vi "Autonomous Independent.vi"() -> ()   [LabVIEW 2019]
doc: "This VI is called when autonomous begins, and will automatically be terminated when autonomous ends. You can carry out timed or sensor driven robot movement independently without needing to return to the caller."
uses:
  <vilib>/Rock Robotics/WPI/Ultrasonic/WPI_UltrasonicRangeUnits.ctl
  <vilib>/Rock Robotics/WPI/Utilities/WPI_GetSetVariantRefNum.vi
  <vilib>/Rock Robotics/Network Tables/NT Read String.vi
  <vilib>/Rock Robotics/Network Tables/NT Write Numeric Array.vi
  <vilib>/Rock Robotics/WPI/Ultrasonic/WPI_SonarSRF04DigitalRefNum Registry Get.vi
  <vilib>/Rock Robotics/WPI/Ultrasonic/WPI_SonarSRF04DigitalGetRange.vi
panel:
  out "Ultrasonic 3":dbl
  out "Ultrasonic 2":dbl
  out "Ultrasonic":dbl
  out "Degrees 2":dbl(knob) scale=0.0..360.0
  out "Degrees":dbl(knob) scale=0.0..360.0
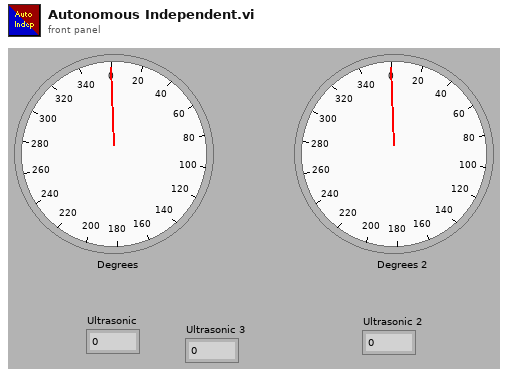
[diagram p1: front panel]
types:
  T1 = typedef "WPI_JoystickDevRef.ctl" = cluster{"Device":T2}
  T2 = typedef "WPI_JoystickDeviceEnum.ctl" = enum16{"USB 0", "USB 1", "USB 2", "USB 3", "USB 4", "USB 5"}
  T3 = typedef "WPI_UltrasonicRangeUnits.ctl" = enum16{"inches", "mm"}
  T4 = typedef "WPI_RobotDriveDevRef.ctl" = cluster{"DevStatus":errorcluster, "Motors[]":T5[], "Square Inputs":bool, "Max Output":dbl}
  T5 = typedef "WPI_MotorControlDeviceRef.ctl" = cluster{"DeviceStatus":errorcluster, "Type":T6, "PWM":cluster{"PWM Channel":T7, "DeadBand":T8}, "CAN":cluster{"Device Number":u8, "SetOutput VI Ref":variant, "GetOutput VI Ref":variant, "Enable VI Ref":variant, "Disable VI Ref":variant, "Data":variant}, "Invert":bool, "DIO PWM":cluster{"PWM \"Enable\" Channel":T7, "DIOChannel":T9, "PWM Rate":dbl}}
  T6 = typedef "WPI_MotorControlType.ctl" = enum16{"PWM", "CAN", "DIO PWM"}
  T7 = typedef "FPGA_DIOPWMChannel.ctl" = enum8{"PWM 0", "PWM 1", "PWM 2", "PWM 3", "PWM 4", "PWM 5", "PWM 6", "PWM 7", "PWM 8", "PWM 9", "PWM MXP 0", "PWM MXP 1", "PWM MXP 2", "PWM MXP 3", "PWM MXP 4", "PWM MXP 5", "PWM MXP 6", "PWM MXP 7", "PWM MXP 8", "PWM MXP 9", "Invalid"}
  T8 = typedef "WPI_PWMDeadband.ctl" = cluster{"Name":string, "maxPositivePwm":i32, "minPositivePwm":i32, "centerPwm":i32, "maxNegativePwm":i32, "minNegativePwm":i32, "angularRange":u16}
  T9 = typedef "FPGA_DIOChannel.ctl" = enum8{"DIO 0", "DIO 1", "DIO 2", "DIO 3", "DIO 4", "DIO 5", "DIO 6", "DIO 7", "DIO 8", "DIO 9", "DIO MXP 0", "DIO MXP 1", "DIO MXP 2", "DIO MXP 3", "DIO MXP 4", "DIO MXP 5", "DIO MXP 6", "DIO MXP 7", "DIO MXP 8", "DIO MXP 9", "DIO MXP 10", "DIO MXP 11", "DIO MXP 12", "DIO MXP 13", "DIO MXP 14", "DIO MXP 15", "SPI Port CS1", "SPI Port CS2", "SPI Port CS3", "SPI Port MISO", "SPI Port MOSI", "Invalid"}
  T10 = typedef "WPI_I2CDevRef.ctl" = cluster{"DevStatus":errorcluster, "Device Address":u8, "Handle":i32, "I2C Bus":T11}
  T11 = typedef "i2c_bus.ctl" = enum16{"I2C On-Board", "I2C MXP", "Invalid"}
  T12 = typedef "WPI_UltrasonicDeviceRef.ctl" = cluster{"DevStatus":errorcluster, "Ping Channel":T9, "Echo Channel":T9, "CntIndex":T13}
  T13 = typedef "FPGA_CounterCtrSystemIndex.ctl" = enum8{"Ctr 0", "Ctr 1", "Ctr 2", "Ctr 3", "Ctr 4", "Ctr 5", "Ctr 6", "Ctr 7", "Invalid"}
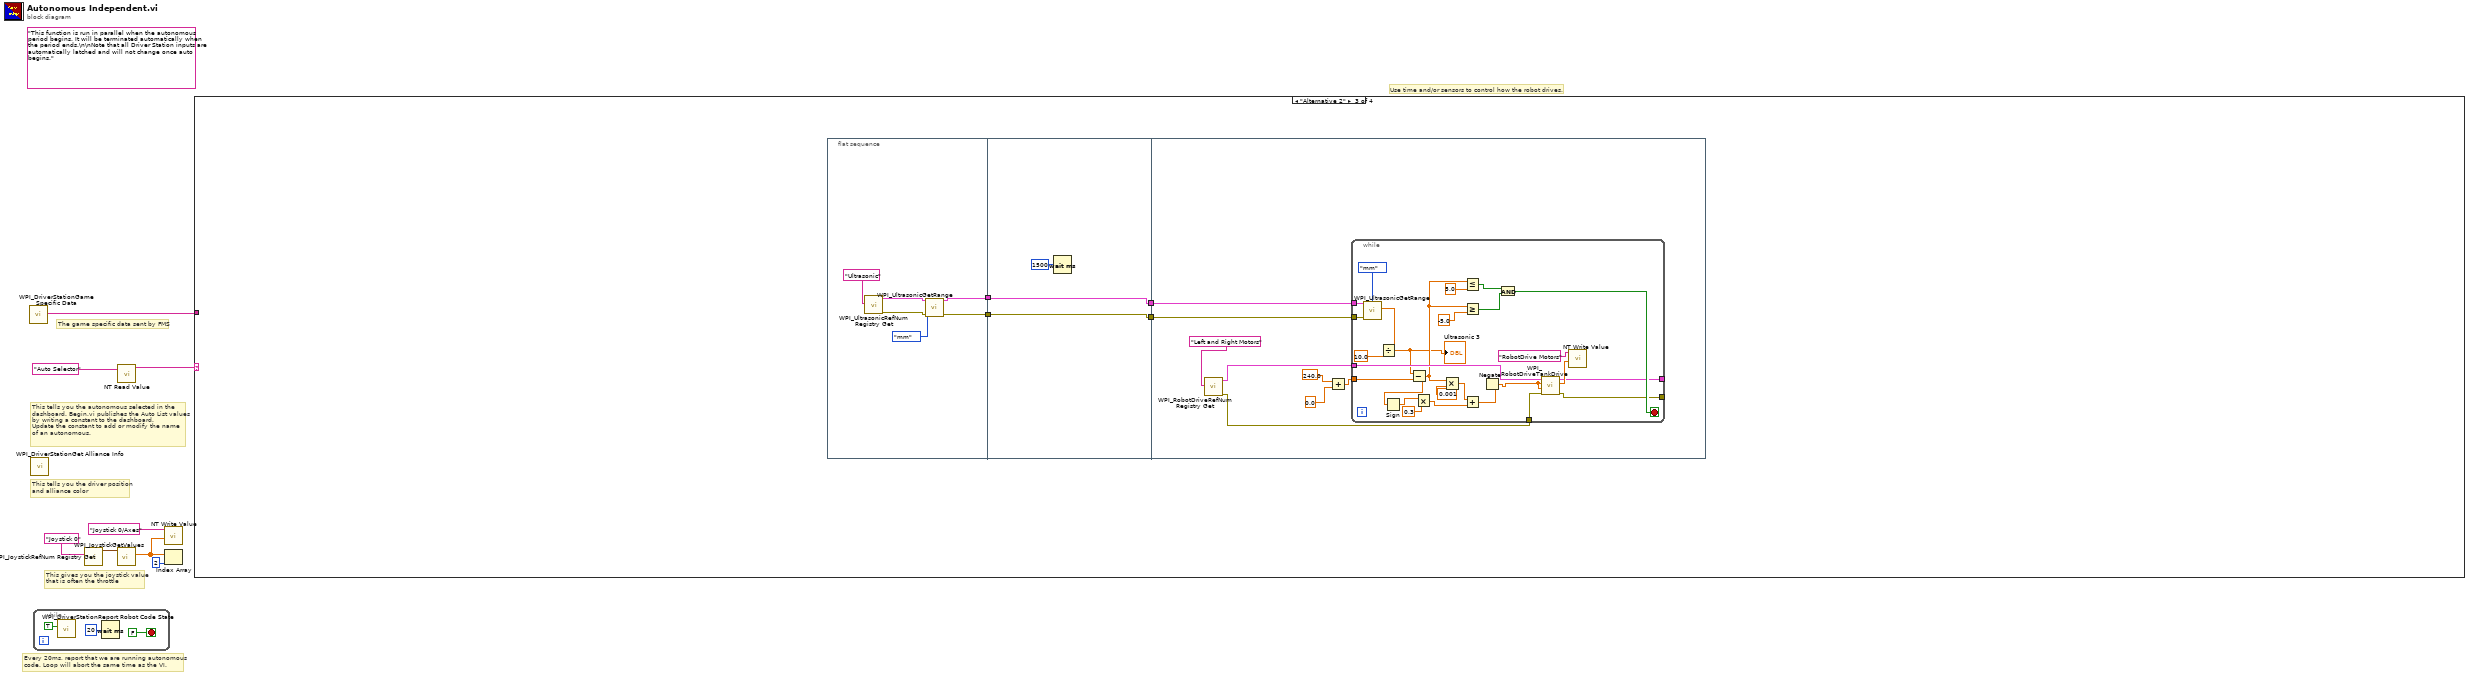
[diagram p0: block diagram]
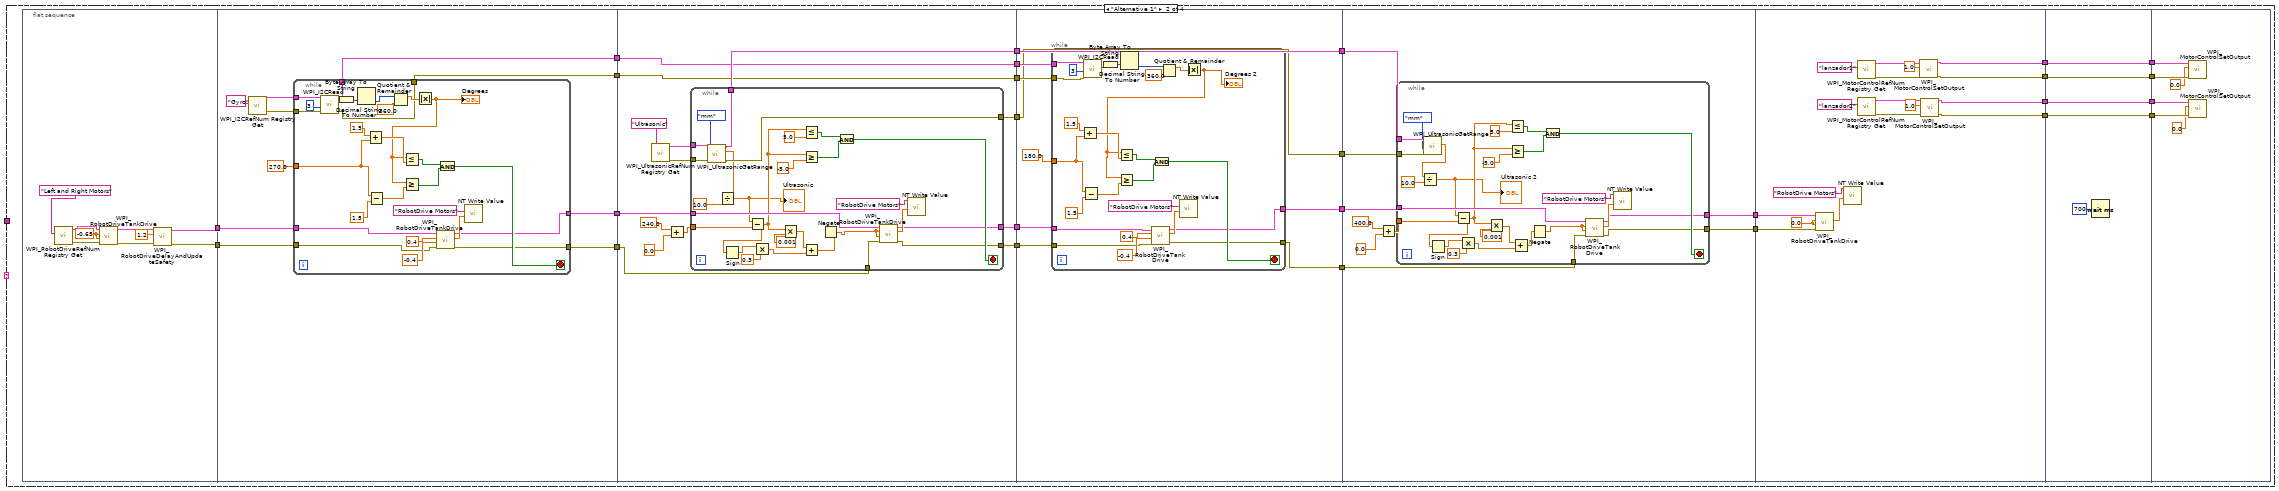
[diagram p3: hidden frame]
diagram:
  (unwired) "This function is run in parallel when the autonomous period begins. It will be terminated automatically when the period ends.\n\nNote that all Driver Station inputs are automatically latched and will not change once auto begins."
  # "The game specific data sent by FMS"
  # "This tells you the autonomous selected in the \ndashboard. Begin.vi publishes the Auto List values\nby writing a constant to the dashboard.\nUpdate the constant to add or modify the name\nof an autonomous."
  # "Every 20ms, report that we are running autonomous\ncode. Loop will abort the same time as the VI."
  # "This gives you the joystick value\nthat is often the throttle"
  # "Use time and/or sensors to control how the robot drives."
  # "This tells you the driver position\nand alliance color"
  n1 = call <vilib>:"WPI_DriverStationGame Specific Data.vi"() -> ("Game Specific Data"=w1:string)  [unwired: 11 in]
  n2 = call <vilib>:"WPI_DriverStationGet Alliance Info.vi"() -> ()  [unwired: 12 out]
  n3 = while {
    stop <- FALSE stop-if-true
    n4 = call <vilib>:"WPI_DriverStationReport Robot Code State.vi"("Autonomous"=TRUE) -> ()  [unwired: 10 in, 1 out]
    n5 = Wait (ms)(milliseconds to wait=u32 20) -> ()  [unwired: 1 out]
  }
  n6 = call <vilib>:"WPI_JoystickRefNum Registry Get.vi"("refnum name"="Joystick 0") -> ("JoystickDevRef"=w7:T1)  [unwired: 1 in, 9 out]
  n7 = call <vilib>:"WPI_JoystickGetValues.vi"("JoystickDevRef"=w7) -> ("Axes"=w3:dbl[])  [unwired: 6 in, 4 out]
  n8 = call-poly <vilib>:"NT Read Value.vi"("Name"="Auto Selector") -> ("String"=w4:string)  [unwired: 9 in, 1 out]
  n9 = call-poly <vilib>:"NT Write Value.vi"("Numeric Array"=w3, "Name"="Joystick 0/Axes") -> ()  [unwired: 9 in, 1 out]
  n10 = Index Array(array=w3, index=2) -> ()  [unwired: 1 out]
  n11 = case shown="\"Alternative 2\"" w4 {
    tunnel: w1 -> [_ _ _ _]
    frame Default {
      # "You can put your main auto here, or you can right-click on the case and make any\nother frame be the default case."
      # "This is the frame that will execute if no selection is made, or if it is not recognized"
    }
    frame "Alternative 1" {
      n12 = flat-sequence {
        tunnel: [w39] -> w15
        tunnel: [w40] -> w14
        tunnel: [w55] -> w37
        tunnel: [w54] -> w36
        tunnel: w15 -> [w50]
        tunnel: w14 -> [w49]
        tunnel: [w48] -> w13
        tunnel: [w47] -> w12
        tunnel: w37 -> [w91]
        tunnel: w36 -> [w90]
        tunnel: [w89] -> w35
        tunnel: [w88] -> w34
        tunnel: [w85] -> w33
        tunnel: [w84] -> w32
        tunnel: [w87] -> w31
        tunnel: [w86] -> w30
        tunnel: w13 -> [w85]
        tunnel: w12 -> [w84]
        tunnel: w35 -> [w134]
        tunnel: w34 -> [w133]
        tunnel: w33 -> [w131]
        tunnel: w32 -> [w130]
        tunnel: [w129] -> w29
        tunnel: [w128] -> w28
        tunnel: [w127] -> w27
        tunnel: w31 -> [w127]
        tunnel: [w126] -> w26
        tunnel: w30 -> [w126]
        tunnel: w29 -> [w168]
        tunnel: w28 -> [w164]
        tunnel: w27 -> [w163]
        tunnel: w26 -> [w162]
        tunnel: [w161] -> w25
        tunnel: [w160] -> w24
        tunnel: w25 -> [w201]
        tunnel: w24 -> [w200]
        tunnel: [w198] -> w23
        tunnel: [w197] -> w22
        tunnel: [w196] -> w21
        tunnel: [w195] -> w20
        tunnel: [w215] -> w19
        tunnel: w23 -> [w215]
        tunnel: [w214] -> w18
        tunnel: w22 -> [w214]
        tunnel: [w213] -> w17
        tunnel: w21 -> [w213]
        tunnel: [w212] -> w16
        tunnel: w20 -> [w212]
        tunnel: w19 -> [w222]
        tunnel: w18 -> [w221]
        tunnel: w17 -> [w220]
        tunnel: w16 -> [w219]
        frame #0 {
          w44 = -0.65 ("Left axis value")
          n13 = call <vilib>:"WPI_RobotDriveRefNum Registry Get.vi"("refnum name"="Left and Right Motors") -> ("error out"=w42:errorcluster, "RobotDriveDevRef"=w43:T4)  [unwired: 9 in]
          n14 = call <vilib>:"WPI_RobotDriveTankDrive.vi"("error in (no error)"=w42, "Right axis value"=w44, "Left axis value"=w44, "RobotDriveDevRef"=w43) -> ("error out"=w45:errorcluster, "RobotDriveDevRef"=w46:T4)  [unwired: 5 in, 1 out]
          n15 = call <vilib>:"WPI_RobotDriveDelayAndUpdateSafety.vi"("error in (no error)"=w45, "Delay (s)"=1.2, "RobotDriveDevRef"=w46) -> ("error out"=w39:errorcluster, "RobotDriveDevRef 2"=w40:T4)  [unwired: 7 in]
        }
        frame #1 {
          n16 = call <vilib>:"WPI_I2CRefNum Registry Get.vi"("refnum name"="Gyro") -> ("error out"=w52:errorcluster, "I2CDevRef"=w51:T10)  [unwired: 9 in]
          n17 = while {
            tunnel: 270.0 ("y") -> [w76]
            tunnel: [w69] -> w55
            tunnel: [w68] -> w54
            tunnel: w52 -> [w65]
            tunnel: w51 -> [w64]
            tunnel: w50 -> [w60]
            tunnel: w49 -> [w59]
            tunnel: [w58] -> w48
            tunnel: [w57] -> w47
            stop <- w79 stop-if-true
            n18 = call <vilib>:"WPI_I2CRead.vi"("error in (no error)"=w65, "I2CBytesToRead"=u8 3, "I2CDevRef"=w64) -> ("error out"=w57:errorcluster, "Data Out"=w62:u8[], "I2CDevRef"=w58:T10)  [unwired: 6 in]
            n19 = Byte Array To String(unsigned byte array=w62) -> (string=w66:string)
            n20 = Decimal String To Number(string=w66) -> (number=w61:i32)  [unwired: 2 in, 1 out]
            n21 = Add(x=1.5 ("y"), y=w76) -> (x+y=w72:dbl)
            n22 = Subtract(x=w76, y=1.5 ("x")) -> (x-y=w73:dbl)
            n23 = Quotient & Remainder(x=w61, y=360.0) -> (x-y*floor(x/y)=w70:dbl)  [unwired: 1 out]
            n24 = Absolute Value(x=w70) -> (abs(x)=w67:dbl)
            "Degrees" <- w67
            n25 = Less Or Equal?(x=w67, y=w72) -> (x <= y?=w74:bool)
            n26 = Greater Or Equal?(x=w67, y=w73) -> (x >= y?=w75:bool)
            n27 = call <vilib>:"WPI_RobotDriveTankDrive.vi"("error in (no error)"=w60, "Right axis value"=-0.4 ("X axis value"), "Left axis value"=0.4 ("X axis value"), "RobotDriveDevRef"=w59) -> ("error out"=w68:errorcluster, "Motor Values"=w83:dbl[], "RobotDriveDevRef"=w69:T4)  [unwired: 5 in]
            n28 = And(x=w74, y=w75) -> (x .and. y?=w79:bool)
            n29 = call-poly <vilib>:"NT Write Value.vi"("Numeric Array"=w83, "Name"="RobotDrive Motors") -> ()  [unwired: 9 in, 1 out]
          }
        }
        frame #2 {
          n30 = call-poly <vilib>:"WPI_UltrasonicRefNum Registry Get.vi"("refnum name"="Ultrasonic") -> ("error out"=w96:errorcluster, "SonarSRF04DevRef"=w95:T12)  [unwired: 9 in]
          n31 = Add(x=240.0 ("y"), y=0.0) -> (x+y=w92:dbl)
          n32 = while {
            tunnel: w96 -> [w107]
            tunnel: w95 -> [w106]
            tunnel: w92 -> [w125]
            tunnel: w91 -> [w120]
            tunnel: w90 -> [w116]
            tunnel: [w109] -> w89
            tunnel: [w108] -> w88
            tunnel: [w104] -> w87
            tunnel: [w103] -> w86
            stop <- w113 stop-if-true
            n33 = call-poly <vilib>:"WPI_UltrasonicGetRange.vi"("error in (no error)"=w107, "Range Units"=WPI_UltrasonicRangeUnits."mm", "SonarSRF04DevRef"=w106) -> ("error out"=w103:errorcluster, "Distance"=w102:dbl, "SonarSRF04DevRef"=w104:T12)  [unwired: 6 in]
            n34 = Divide(x=w102, y=10.0) -> (x/y=w100:dbl)
            "Ultrasonic" <- w100
            n35 = Subtract(x=w100, y=w125) -> (x-y=w110:dbl)
            n36 = Sign(1:w110) -> (0:w119:dbl)
            n37 = Multiply(x=w119, y=0.3) -> (x*y=w117:dbl)
            n38 = Multiply(x=w110, y=0.001) -> (x*y=w123:dbl)
            n39 = Less Or Equal?(x=w110, y=5.0 ("x")) -> (x <= y?=w115:bool)
            n40 = Greater Or Equal?(x=w110, y=-5.0 ("x")) -> (x >= y?=w114:bool)
            n41 = Add(x=w123, y=w117) -> (x+y=w99:dbl)
            n42 = Negate(x=w99) -> (-x=w98:dbl)
            n43 = And(x=w115, y=w114) -> (x .and. y?=w113:bool)
            n44 = call <vilib>:"WPI_RobotDriveTankDrive.vi"("error in (no error)"=w116, "Right axis value"=w98, "Left axis value"=w98, "RobotDriveDevRef"=w120) -> ("error out"=w109:errorcluster, "Motor Values"=w122:dbl[], "RobotDriveDevRef"=w108:T4)  [unwired: 5 in]
            n45 = call-poly <vilib>:"NT Write Value.vi"("Numeric Array"=w122, "Name"="RobotDrive Motors") -> ()  [unwired: 9 in, 1 out]
          }
        }
        frame #3 {
          n46 = while {
            tunnel: w133 -> [w155]
            tunnel: w134 -> [w154]
            tunnel: 180.0 ("y") -> [w150]
            tunnel: [w143] -> w129
            tunnel: [w142] -> w128
            tunnel: w131 -> [w138]
            tunnel: w130 -> [w137]
            stop <- w153 stop-if-true
            n47 = Add(x=1.5 ("y"), y=w150) -> (x+y=w146:dbl)
            n48 = Subtract(x=w150, y=1.5 ("x")) -> (x-y=w147:dbl)
            n49 = call <vilib>:"WPI_I2CRead.vi"("error in (no error)"=w137, "I2CBytesToRead"=u8 3, "I2CDevRef"=w138) -> ("Data Out"=w139:u8[])  [unwired: 6 in, 2 out]
            n50 = Byte Array To String(unsigned byte array=w139) -> (string=w141:string)
            n51 = Decimal String To Number(string=w141) -> (number=w136:i32)  [unwired: 2 in, 1 out]
            n52 = call <vilib>:"WPI_RobotDriveTankDrive.vi"("error in (no error)"=w154, "Right axis value"=-0.4 ("X axis value"), "Left axis value"=0.4 ("X axis value"), "RobotDriveDevRef"=w155) -> ("error out"=w142:errorcluster, "Motor Values"=w159:dbl[], "RobotDriveDevRef"=w143:T4)  [unwired: 5 in]
            n53 = Quotient & Remainder(x=w136, y=360.0) -> (x-y*floor(x/y)=w144:dbl)  [unwired: 1 out]
            n54 = call-poly <vilib>:"NT Write Value.vi"("Numeric Array"=w159, "Name"="RobotDrive Motors") -> ()  [unwired: 9 in, 1 out]
            n55 = Absolute Value(x=w144) -> (abs(x)=w135:dbl)
            "Degrees 2" <- w135
            n56 = Less Or Equal?(x=w135, y=w146) -> (x <= y?=w148:bool)
            n57 = Greater Or Equal?(x=w135, y=w147) -> (x >= y?=w149:bool)
            n58 = And(x=w148, y=w149) -> (x .and. y?=w153:bool)
          }
        }
        frame #4 {
          n59 = Add(x=400.0 ("y"), y=0.0) -> (x+y=w165:dbl)
          n60 = while {
            tunnel: w162 -> [w176]
            tunnel: w163 -> [w175]
            tunnel: w165 -> [w194]
            tunnel: w168 -> [w189]
            tunnel: w164 -> [w185]
            tunnel: [w178] -> w161
            tunnel: [w177] -> w160
            stop <- w182 stop-if-true
            n61 = call-poly <vilib>:"WPI_UltrasonicGetRange.vi"("error in (no error)"=w176, "Range Units"=WPI_UltrasonicRangeUnits."mm", "SonarSRF04DevRef"=w175) -> ("Distance"=w173:dbl)  [unwired: 6 in, 2 out]
            n62 = Divide(x=w173, y=10.0) -> (x/y=w171:dbl)
            "Ultrasonic 2" <- w171
            n63 = Subtract(x=w171, y=w194) -> (x-y=w179:dbl)
            n64 = Sign(1:w179) -> (0:w188:dbl)
            n65 = Multiply(x=w188, y=0.3) -> (x*y=w186:dbl)
            n66 = Multiply(x=w179, y=0.001) -> (x*y=w192:dbl)
            n67 = Less Or Equal?(x=w179, y=5.0 ("x")) -> (x <= y?=w184:bool)
            n68 = Greater Or Equal?(x=w179, y=-5.0 ("x")) -> (x >= y?=w183:bool)
            n69 = Add(x=w192, y=w186) -> (x+y=w170:dbl)
            n70 = Negate(x=w170) -> (-x=w169:dbl)
            n71 = And(x=w184, y=w183) -> (x .and. y?=w182:bool)
            n72 = call <vilib>:"WPI_RobotDriveTankDrive.vi"("error in (no error)"=w185, "Right axis value"=w169, "Left axis value"=w169, "RobotDriveDevRef"=w189) -> ("error out"=w177:errorcluster, "Motor Values"=w191:dbl[], "RobotDriveDevRef"=w178:T4)  [unwired: 5 in]
            n73 = call-poly <vilib>:"NT Write Value.vi"("Numeric Array"=w191, "Name"="RobotDrive Motors") -> ()  [unwired: 9 in, 1 out]
          }
        }
        frame #5 {
          w199 = 0.0 ("Left axis value")
          n74 = call <vilib>:"WPI_RobotDriveTankDrive.vi"("error in (no error)"=w200, "Right axis value"=w199, "Left axis value"=w199, "RobotDriveDevRef"=w201) -> ("Motor Values"=w203:dbl[])  [unwired: 5 in, 2 out]
          n75 = call-poly <vilib>:"NT Write Value.vi"("Numeric Array"=w203, "Name"="RobotDrive Motors") -> ()  [unwired: 9 in, 1 out]
          n76 = call <vilib>:"WPI_MotorControlRefNum Registry Get.vi"("refnum name"="lanzador1") -> ("error out"=w210:errorcluster, "MotorControlDevRef"=w211:T5)  [unwired: 9 in]
          n77 = call <vilib>:"WPI_MotorControlRefNum Registry Get.vi"("refnum name"="lanzador2") -> ("error out"=w206:errorcluster, "MotorControlDevRef"=w207:T5)  [unwired: 9 in]
          n78 = call <vilib>:"WPI_MotorControlSetOutput.vi"("error in (no error)"=w210, "Output"=1.0, "MotorControlDevRef"=w211) -> ("error out"=w195:errorcluster, "MotorControlDevRef"=w198:T5)  [unwired: 6 in, 1 out]
          n79 = call <vilib>:"WPI_MotorControlSetOutput.vi"("error in (no error)"=w206, "Output"=1.0, "MotorControlDevRef"=w207) -> ("error out"=w196:errorcluster, "MotorControlDevRef"=w197:T5)  [unwired: 6 in, 1 out]
        }
        frame #6 {
          n80 = Wait (ms)(milliseconds to wait=u32 700) -> ()  [unwired: 1 out]
        }
        frame #7 {
          n81 = call <vilib>:"WPI_MotorControlSetOutput.vi"("error in (no error)"=w219, "Output"=0.0, "MotorControlDevRef"=w222) -> ()  [unwired: 6 in, 3 out]
          n82 = call <vilib>:"WPI_MotorControlSetOutput.vi"("error in (no error)"=w220, "Output"=0.0, "MotorControlDevRef"=w221) -> ()  [unwired: 6 in, 3 out]
        }
      }
    }
    frame "Alternative 2" {
      n83 = flat-sequence {
        tunnel: [w230] -> w224
        tunnel: [w231] -> w223
        tunnel: [w234] -> w226
        tunnel: [w233] -> w225
        tunnel: w224 -> [w234]
        tunnel: w223 -> [w233]
        tunnel: w226 -> [w237]
        tunnel: w225 -> [w236]
        frame #0 {
          n84 = call-poly <vilib>:"WPI_UltrasonicRefNum Registry Get.vi"("refnum name"="Ultrasonic") -> ("error out"=w227:errorcluster, "SonarSRF04DevRef"=w228:T12)  [unwired: 9 in]
          n85 = call-poly <vilib>:"WPI_UltrasonicGetRange.vi"("error in (no error)"=w227, "Range Units"=WPI_UltrasonicRangeUnits."mm", "SonarSRF04DevRef"=w228) -> ("error out"=w230:errorcluster, "SonarSRF04DevRef"=w231:T12)  [unwired: 6 in, 1 out]
        }
        frame #1 {
          n86 = Wait (ms)(milliseconds to wait=u32 1500) -> ()  [unwired: 1 out]
        }
        frame #2 {
          n87 = call <vilib>:"WPI_RobotDriveRefNum Registry Get.vi"("refnum name"="Left and Right Motors") -> ("error out"=w238:errorcluster, "RobotDriveDevRef"=w239:T4)  [unwired: 9 in]
          n88 = Add(x=240.0 ("y"), y=0.0) -> (x+y=w241:dbl)
          n89 = while {
            tunnel: w241 -> [w269]
            tunnel: w239 -> [w264]
            tunnel: w238 -> [w260]
            tunnel: [w253] -> _
            tunnel: [w252] -> _
            tunnel: w237 -> [w245]
            tunnel: w236 -> [w244]
            stop <- w257 stop-if-true
            n90 = call-poly <vilib>:"WPI_UltrasonicGetRange.vi"("error in (no error)"=w245, "Range Units"=WPI_UltrasonicRangeUnits."mm", "SonarSRF04DevRef"=w244) -> ("Distance"=w250:dbl)  [unwired: 6 in, 2 out]
            n91 = Divide(x=w250, y=10.0) -> (x/y=w248:dbl)
            "Ultrasonic 3" <- w248
            n92 = Subtract(x=w248, y=w269) -> (x-y=w254:dbl)
            n93 = Sign(1:w254) -> (0:w263:dbl)
            n94 = Multiply(x=w263, y=0.3) -> (x*y=w261:dbl)
            n95 = Multiply(x=w254, y=0.001) -> (x*y=w267:dbl)
            n96 = Less Or Equal?(x=w254, y=5.0 ("x")) -> (x <= y?=w259:bool)
            n97 = Greater Or Equal?(x=w254, y=-5.0 ("x")) -> (x >= y?=w258:bool)
            n98 = Add(x=w267, y=w261) -> (x+y=w247:dbl)
            n99 = Negate(x=w247) -> (-x=w246:dbl)
            n100 = And(x=w259, y=w258) -> (x .and. y?=w257:bool)
            n101 = call <vilib>:"WPI_RobotDriveTankDrive.vi"("error in (no error)"=w260, "Right axis value"=w246, "Left axis value"=w246, "RobotDriveDevRef"=w264) -> ("error out"=w253:errorcluster, "Motor Values"=w266:dbl[], "RobotDriveDevRef"=w252:T4)  [unwired: 5 in]
            n102 = call-poly <vilib>:"NT Write Value.vi"("Numeric Array"=w266, "Name"="RobotDrive Motors") -> ()  [unwired: 9 in, 1 out]
          }
        }
      }
    }
    frame "Your Turn" {
    }
  }
